vi "Read Graph Data.vi"(11 "IMD in":refnum<class "IMD.lvclass">) -> (2 "Graph Data":cluster{"Array":dbl[], "Array":dbl[]}[](array[cluster]), 3 "IMD out":refnum<class "IMD.lvclass">)   [LabVIEW 2020, in "IMD.lvclass"]
uses:
  IMD.lvclass
  IMD.lvclass/IMD.ctl
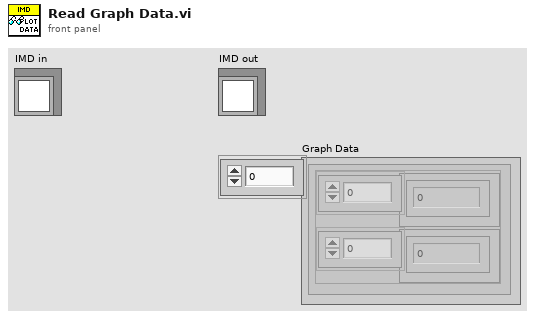
[diagram p1: front panel]
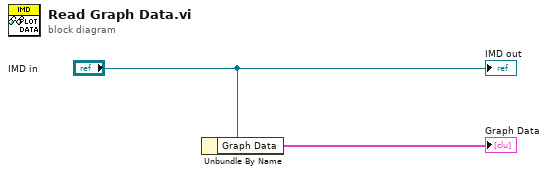
[diagram p0: block diagram]
diagram:
  n1 = Unbundle By Name("IMD in") -> ("Graph Data"=→"Graph Data":cluster{"Array":dbl[], "Array":dbl[]}[])
  "IMD out" <- "IMD in"
